vi "TW Replace Missing Denpendency VIs - Custom gRPC Service Core.vi"(8 "error in":errorcluster, 9 "gRPC Service Name":string, 10 "Project Path":path, 11 "VI Refnum":refnum<vi>) -> (0 "error out":errorcluster)   [LabVIEW 2021, in "Plugin Generator.lvlib"]
uses:
  Plugin Generator.lvlib
  <vilib>/Utility/traverseref.llb/TRef TravTarget.ctl
  <vilib>/Utility/traverseref.llb/VI Scripting - Traverse.lvlib
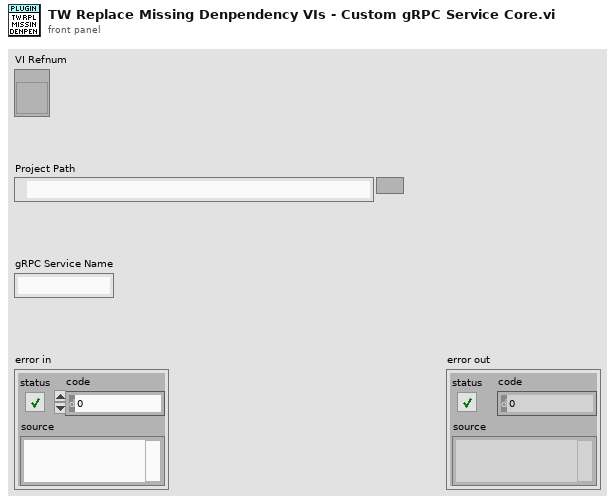
[diagram p1: front panel]
types:
  T1 = typedef "TRef TravTarget.ctl" = enum16{"FP", "BD", "Other"}
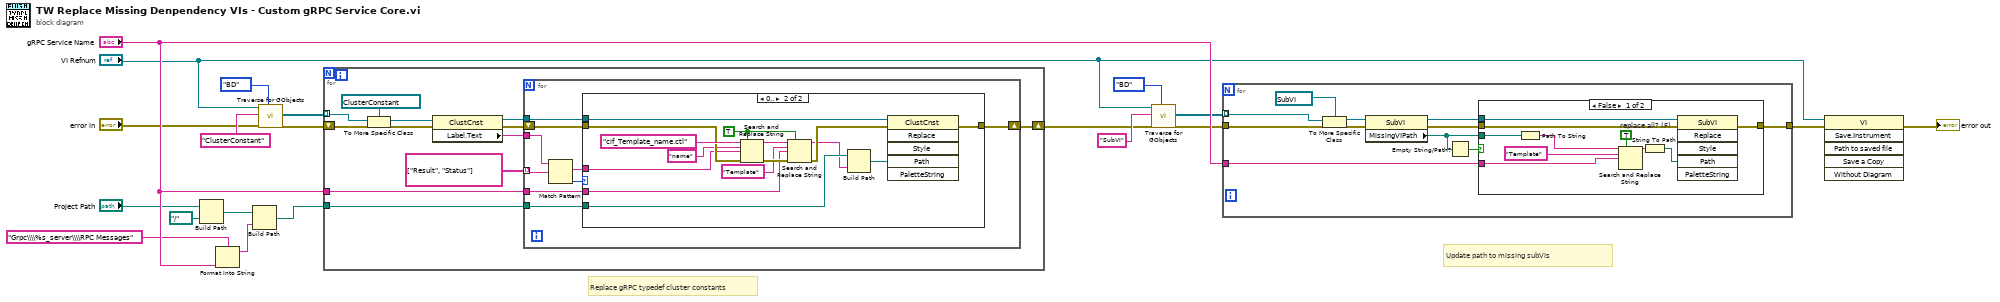
[diagram p0: block diagram]
diagram:
  # "Update path to missing subVIs"
  # "Replace gRPC typedef cluster constants"
  n1 = Build Path(base path="Project Path", name or relative path=path "../..") -> (appended path=w13:path)
  n2 = Format Into String(format string="Grpc\\\\%s_server\\\\RPC Messages" ("Class Name"), "gRPC Service Name") -> (resulting string=w16:string)  [unwired: 2 in, 1 out]
  n3 = Build Path(base path=w13, name or relative path=w16) -> (appended path=w4:path)
  n4 = call <vilib>:"Traverse for GObjects.vi"("Traverse Target"=TRef_TravTarget."BD", "error in (no error)"="error in", "Class Name"="ClusterConstant", "VI Refnum"="VI Refnum") -> ("error out"=w10:errorcluster, "References"=w19:refnum<vi>[])  [unwired: 4 in, 2 out]
  n5 = for {
    tunnel: w19 -> [w32] mode=indexing
    tunnel: "gRPC Service Name" -> [w25]
    shift-right: [w27] -> w5
    shift-left: w10 -> [w23]
    tunnel: w4 -> [w22]
    n6 = To More Specific Class(target class=refnum<vi> refnum ("x"), reference=w32, error in=w23) -> (specific class reference=w26:refnum<vi>, error out=w30:errorcluster)
    n7 = property class="ClustCnst"(reference=w26, error in=w30) -> (reference out=w28:refnum<vi>, error out=w29:errorcluster, "Label.Text"=w24:string)
    n8 = for {
      tunnel: w28 -> [w40]
      tunnel: w25 -> [w37]
      tunnel: w24 -> [w36]
      tunnel: w22 -> [w38]
      shift-right: [w39] -> w27
      shift-left: w29 -> [w41]
      tunnel: string[] ["Result", "Status"] -> [w34] mode=indexing
      n9 = Match Pattern(string=w36, regular expression=w34) -> (match substring=w33:string, offset past match=w35:i32)  [unwired: 1 in, 2 out]
      n10 = case shown="0.." w35 {
        tunnel: w41 -> [w42 w49]
        tunnel: w40 -> [_ w57]
        tunnel: [w42 w56] -> w39
        tunnel: w38 -> [_ w55]
        tunnel: w37 -> [_ w45]
        tunnel: w33 -> [_ w44]
        frame Default {
        }
        frame 0.. {
          w51 = TRUE ("replace all? (F)")
          n11 = Search and Replace String(replace all?=w51, input string="cif_Template_name.ctl", search string="name", replace string=w44, error in=w49) -> (result string=w52:string, error out=w50:errorcluster)  [unwired: 3 in, 2 out]
          n12 = Search and Replace String(replace all?=w51, input string=w52, search string="Template", replace string=w45, error in=w50) -> (result string=w47:string, error out=w48:errorcluster)  [unwired: 3 in, 2 out]
          n13 = Build Path(base path=w55, name or relative path=w47) -> (appended path=w54:path)
          n14 = invoke class="ClustCnst" method="Replace"(reference=w57, error in=w48, "Path"=w54) -> (error out=w56:errorcluster)  [unwired: 3 in, 5 out]
        }
      }
    }
  }
  n15 = call <vilib>:"Traverse for GObjects.vi"("Traverse Target"=TRef_TravTarget."BD", "error in (no error)"=w5, "Class Name"="SubVI", "VI Refnum"="VI Refnum") -> ("error out"=w6:errorcluster, "References"=w7:refnum<vi>[])  [unwired: 4 in, 2 out]
  n16 = for {
    tunnel: w7 -> [w60] mode=indexing
    tunnel: "gRPC Service Name" -> [w65]
    tunnel: w6 -> [w63]
    tunnel: [w58] -> w11
    n17 = To More Specific Class(target class=refnum<vi> refnum ("x"), reference=w60, error in=w63) -> (specific class reference=w61:refnum<vi>, error out=w59:errorcluster)
    n18 = property class="SubVI"(reference=w61, error in=w59) -> (reference out=w67:refnum<vi>, error out=w64:errorcluster, "MissingVIPath"=w66:path)
    n19 = Empty String/Path?(string/path=w66) -> (empty?=w68:bool)
    n20 = case shown="False" w68 {
      tunnel: w67 -> [w78 _]
      tunnel: w66 -> [w76 _]
      tunnel: w65 -> [w72 _]
      tunnel: w64 -> [w70 w79]
      tunnel: [w69 w79] -> w58
      frame False {
        w71 = TRUE  # replace all? (F)
        n21 = Path To String(path=w76) -> (string=w77:string)
        n22 = Search and Replace String(replace all?=w71, input string=w77, search string="Template", replace string=w72) -> (result string=w74:string)  [unwired: 4 in, 3 out]
        n23 = String To Path(string=w74) -> (path=w73:path)
        n24 = invoke class="SubVI" method="Replace"(reference=w78, error in=w70, "Path"=w73) -> (error out=w69:errorcluster)  [unwired: 3 in, 5 out]
      }
      frame True {
      }
    }
  }
  n25 = invoke class="VI" method="Save.Instrument"(reference="VI Refnum", error in=w11) -> (error out=→"error out":errorcluster)  [unwired: 4 in, 5 out]
